vi "Copy Linked List Attributes.vi"(7 "Sink Linked List ID":string, 8 "error in (no error)":errorcluster, 10 "Source Linked List ID":string, 11 "Linked List in":refnum<class "Linked List.lvclass">) -> (0 "error out":errorcluster, 3 "Linked List out":refnum<class "Linked List.lvclass">)   [LabVIEW 2020, in "Linked Lists.lvlib" / "Linked List.lvclass"]
uses:
  <vilib>/gpm_packages/@cs/linked-list/Source/Linked List/Linked List/Linked List.lvclass
  <vilib>/gpm_packages/@cs/linked-list/Source/Linked List/Linked List Definition/Linked List Definition.lvclass
  <vilib>/gpm_packages/@cs/linked-list/Source/Linked List/Linked List/Linked List.lvclass/Linked List.ctl
  <vilib>/gpm_packages/@cs/lookup-table/Source/LookupTable/LookupTable.lvclass/LookupTable.ctl
  8f41429e-3381-47c5-98a2-27ef3cc9fac2.vi
  <vilib>/gpm_packages/@cs/lookup-table/Source/LookupTable/Read Table Reference.vi
  8f41429e-3381-47c5-98a2-27ef3cc9fac2.vi/7d7783b1-84c6-4422-8328-addec0ded6f9.vi
  <vilib>/gpm_packages/@cs/lookup-table/Source/LookupTable/LookupTable.lvclass
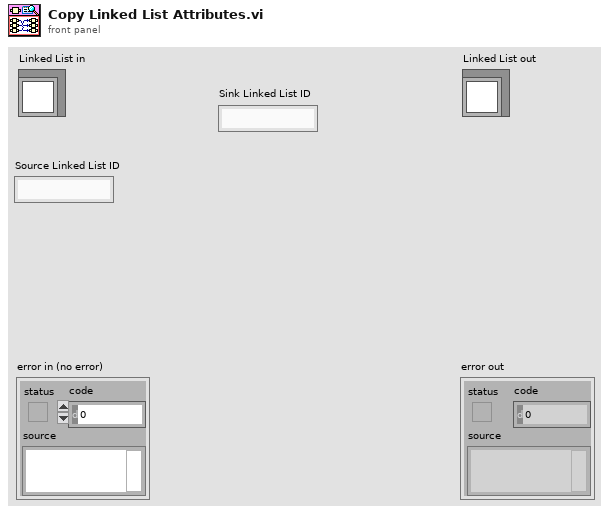
[diagram p1: front panel]
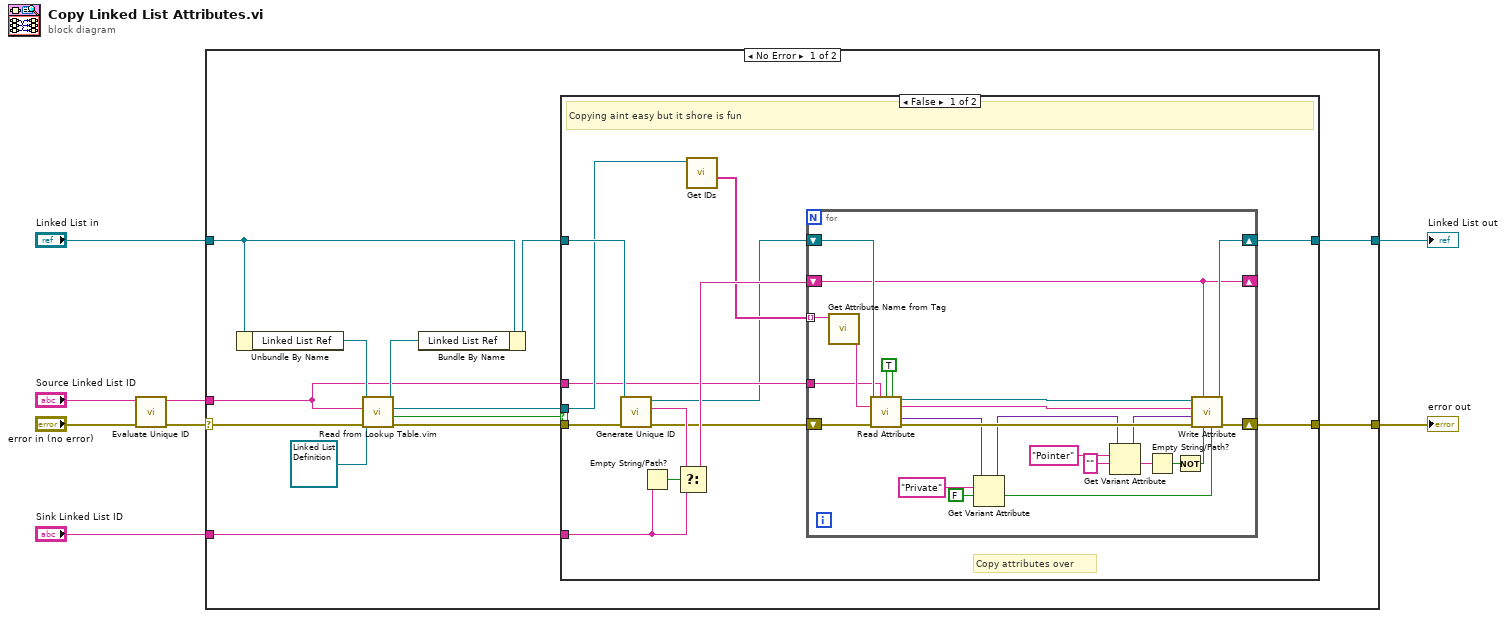
[diagram p0: block diagram]
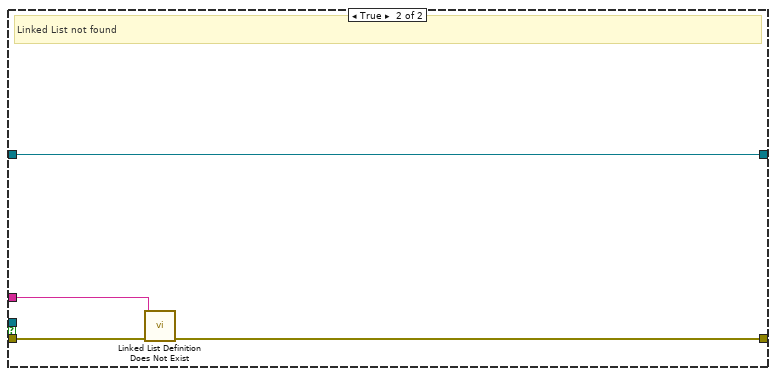
[diagram p2: hidden frame]
diagram:
  n1 = call <vilib>:"Evaluate Unique ID.vi"("error in (no error)"="error in (no error)", "Unique ID"="Source Linked List ID") -> ("error out"=w8:errorcluster, "Unique ID Out"=w7:string)  [unwired: 8 in]
  n2 = case shown="No Error" w8 {
    selector: w8 -> [w19 w62]
    tunnel: w7 -> [w9 _]
    tunnel: "Linked List in" -> [w14 w63]
    tunnel: "Sink Linked List ID" -> [w12 _]
    tunnel: [w11 w63] -> w2
    tunnel: [w10 w62] -> w1
    frame No Error {
      n3 = Unbundle By Name(w14) -> ("Linked List Ref"=w21:refnum<data-value>)
      n4 = call "Read from Lookup Table.vim"("error in (no error)"=w19, "Type"=refnum<class "Linked List Definition.lvclass"> refnum ("Linked List.lvlib:Linked List Definition.lvclass"), "Item Name"=w9, "LookupTable Reference"=w21) -> ("error out"=w17:errorcluster, "Not Found?"=w18:bool, "Value"=w16:refnum<class "Linked List Definition.lvclass">, "LookupTable Reference Out"=w15:refnum<data-value>)  [unwired: 4 in]
      n5 = Bundle By Name(cluster=w14, "Linked List Ref"=w15) -> (w13:refnum<class "Linked List.lvclass">)
      n6 = case shown="False" w18 {
        tunnel: w17 -> [w33 w60]
        tunnel: w16 -> [w28 _]
        tunnel: w13 -> [w34 w61]
        tunnel: w12 -> [w31 _]
        tunnel: [w23 w61] -> w11
        tunnel: [w22 w59] -> w10
        tunnel: w9 -> [w27 w58]
        frame False {
          # "Copy attributes over"
          # "Copying aint easy but it shore is fun"
          n7 = call <vilib>:"Generate Unique ID.vi"("error in (no error)"=w33, "Linked List in"=w34) -> ("error out"=w24:errorcluster, "ID"=w30:string, "Linked List out"=w25:refnum<class "Linked List.lvclass">)  [unwired: 7 in]
          n8 = Empty String/Path?(string/path=w31) -> (empty?=w32:bool)
          n9 = Select(t=w30, s=w32, f=w31) -> (s? t:f=w29:string)
          n10 = call <vilib>:"Get IDs.vi"("Linked List Definition in"=w28) -> ("Data IDs"=w26:string[])  [unwired: 8 in, 2 out]
          n11 = for {
            tunnel: w27 -> [w53]
            shift-right: [w50] -> w22
            shift-left: w24 -> [w57]
            shift-right: [w49] -> w23
            shift-left: w25 -> [w56]
            shift-right: [w48] -> _
            shift-left: w29 -> [w48]
            tunnel: w26 -> [w55] mode=indexing
            w35 = TRUE ("Include Private?")
            n12 = call <vilib>:"Get Attribute Name from Tag.vi"("Tag"=w55) -> ("Attribute Name"=w54:string)  [unwired: 8 in, 2 out]
            n13 = call-dynamic "Read Attribute.vi"("Linked List in"=w56, "Linked List ID"=w53, "Include Private?"=w35, "Flatten Pointer?"=w35, "Attribute Name"=w54, "error in (no error)"=w57) -> ("Linked List out"=w52:refnum<class "Linked List.lvclass">, "Attribute Name out"=w47:string, "Attribute"=w39:variant, "error out"=w51:errorcluster)  [unwired: 4 in, 2 out]
            n14 = Get Variant Attribute(Variant=w39, name="Private", default value (empty Variant)=FALSE) -> (duplicate Variant=w38:variant, value=w36:bool)  [unwired: 1 in, 2 out]
            n15 = Get Variant Attribute(Variant=w38, name="Pointer", default value (empty Variant)="") -> (duplicate Variant=w46:variant, value=w43:string)  [unwired: 1 in, 2 out]
            n16 = Empty String/Path?(string/path=w43) -> (empty?=w42:bool)
            n17 = Not(x=w42) -> (.not. x?=w41:bool)
            n18 = call-dynamic "Write Attribute.vi"("Private?"=w36, "Pointer?"=w41, "Linked List ID"=w48, "error in (no error)"=w51, "Attribute"=w46, "Attribute Name"=w47, "Linked List in"=w52) -> ("error out"=w50:errorcluster, "Linked List out"=w49:refnum<class "Linked List.lvclass">)  [unwired: 1 in, 2 out]
          }
        }
        frame True {
          # "Linked List not found"
          n19 = call <vilib>:"Linked List Definition Does Not Exist.vi"("Error In"=w60, "Unique ID"=w58) -> ("Error Out"=w59:errorcluster)  [unwired: 9 in]
        }
      }
    }
    frame Error {
    }
  }
  "error out" <- w1
  "Linked List out" <- w2
